vi "Read Signal.vi"(8 "error in (no error)":errorcluster, 10 "Rx Signal In":string, 11 "CAN in":refnum<class "CAN.lvclass">) -> (0 "error out":errorcluster, 2 "Signal out":dbl=nan, 3 "CAN out":refnum<class "CAN.lvclass">)   [LabVIEW 2019, in "CAN.lvclass"]
uses:
  CAN.lvclass
  CAN.lvclass/CAN.ctl
  <vilib>/JDP Science/JSONtext/Next JSON Value.vi
  <vilib>/JDP Science/JSONtext/String Subset.vi
  <vilib>/JDP Science/JSONtext/Parsing/Advance past next JSON Value (inlined COPY).vi
  <vilib>/JDP Science/JSONtext/Parsing/Advance past whitespace.vi
  <vilib>/JDP Science/JSONtext/Parsing/Advance past String.vi
  <vilib>/JDP Science/JSONtext/Parsing/Advance past Number.vi
  <vilib>/JDP Science/JSONtext/Parsing/Advance past Line Ending.vi
  <vilib>/xnet/xnet.llb/XNET Read (Signal Single-point).vi
  <vilib>/JDP Science/JSONtext/Parsing/Parse Full Path or Item Name.vi
  <vilib>/JDP Science/JSONtext/Parsing/Advance past Array.vi
  <vilib>/JDP Science/JSONtext/Parsing/Advance past Object.vi
  <vilib>/JDP Science/JSONtext/support/Error Cluster From Code.vi
  <vilib>/JDP Science/JSONtext/Offset/Find Item Locations by Path.vi
  <vilib>/JDP Science/JSONtext/JSONtext.lvlib
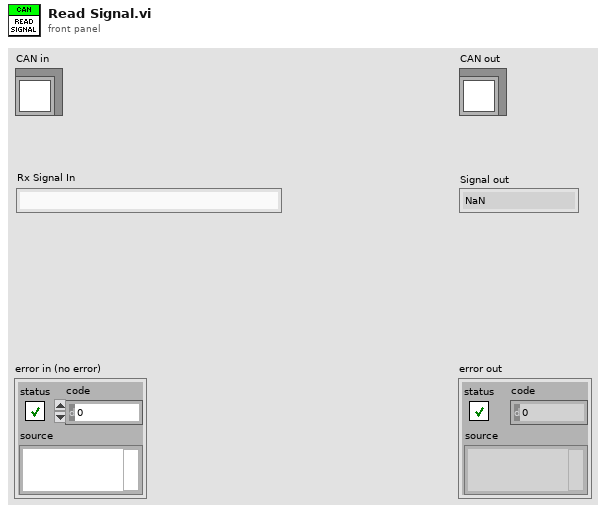
[diagram p1: front panel]
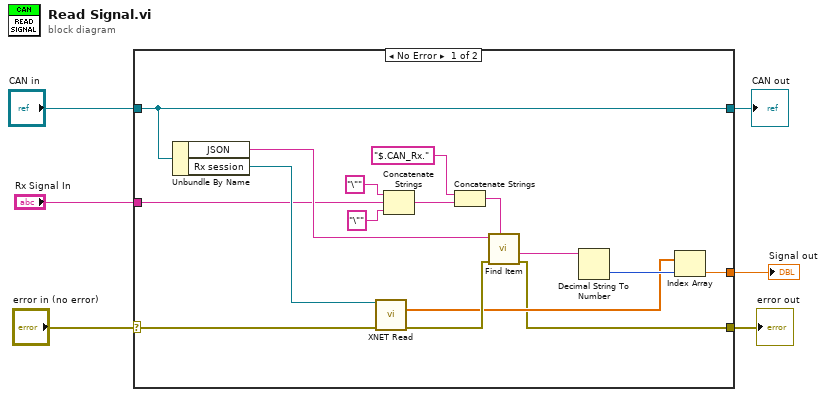
[diagram p0: block diagram]
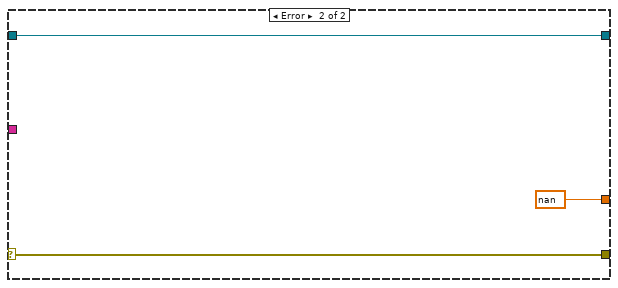
[diagram p2: hidden frame]
diagram:
  n1 = case shown="No Error" "error in (no error)" {
    selector: "error in (no error)" -> [w11 w25]
    tunnel: [w10 w25] -> w5
    tunnel: [w9 w24] -> w3
    tunnel: "CAN in" -> [w9 w24]
    tunnel: "Rx Signal In" -> [w8 _]
    tunnel: [w7 nan] -> w1
    frame No Error {
      n2 = Unbundle By Name(w9) -> ("JSON"=w16:string, "Rx session"=w12:refnum<k21>)
      n3 = call-poly <vilib>:"XNET Read.vi"("session in"=w12, "error in (no error)"=w11) -> ("data"=w13:dbl[], "error out"=w17:errorcluster)  [unwired: 12 out]
      n4 = Concatenate Strings("\"" ("string"), w8, "\"" ("string")) -> (w22:string)
      n5 = Concatenate Strings("$.CAN_Rx." ("$Path or Item Name"), w22) -> (w15:string)
      n6 = call <vilib>:"Find Item.vi"("$Path or Item Name"=w15, "error in (no error)"=w17, "JSON"=w16) -> ("error out"=w10:errorcluster, "<JSON>"=w19:string)  [unwired: 5 in, 2 out]
      n7 = Decimal String To Number(string=w19) -> (number=w18:i32)  [unwired: 2 in, 1 out]
      n8 = Index Array(array=w13, index=w18) -> (element=w7:dbl)
    }
    frame Error {
    }
  }
  "error out" <- w5
  "CAN out" <- w3
  "Signal out" <- w1
